vi "Shox-Total Pulse Width.vi"(1 "Shox":T1={"Rate (pps)"=0.0, "Polarity"=enum."POS", "dB Attenuation"=0.0, "Mode"=enum."Free Run", "Duration (ms)"=0.0, "Burst rate (Hz)"=0.0, "Pulse width (us)"=0.0, "Offset (ms)"=0.0, "Persist"=FALSE, "Sync"=FALSE}) -> (0 "Total pulse width (ms)":dbl)   [LabVIEW 2020]
uses:
  Cochlear Function Test Suite/LV Source/Measurement Sequence VIs/TypeDefs/Pulse Params XCtl/Data.ctl
  Pulse Polarity.ctl
  Cochlear Function Test Suite/LV Source/Measurement Sequence VIs/TypeDefs/Pulse Params XCtl/Shox Mode Enum.ctl
  Cochlear Function Test Suite/LV Source/Measurement Sequence VIs/TypeDefs/Pulse Params XCtl/MS-Pulse Params.xctl
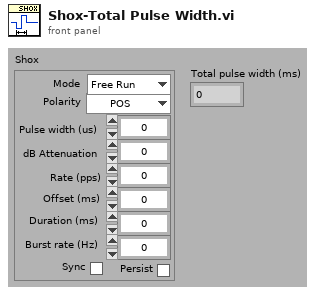
[diagram p1: front panel]
types:
  T1 = typedef "MS-Pulse Params.xctl/Data.ctl" = cluster{"Rate (pps)":dbl, "Polarity":T2, "dB Attenuation":dbl, "Mode":T3, "Duration (ms)":dbl, "Burst rate (Hz)":dbl, "Pulse width (us)":dbl, "Offset (ms)":dbl, "Persist":bool, "Sync":bool}
  T2 = typedef "Pulse Polarity.ctl" = enum16{"POS", "NEG", "POS-NEG", "NEG-POS"}
  T3 = typedef "Shox Mode Enum.ctl" = enum16{"OFF", "Free Run", "Bursted"}
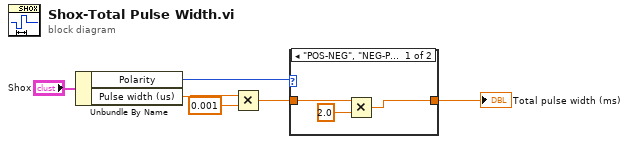
[diagram p0: block diagram]
diagram:
  n1 = Unbundle By Name("Shox") -> ("Polarity"=w4:T2, "Pulse width (us)"=w3:dbl)
  n2 = Multiply(x=w3, y=0.001) -> (x*y=w2:dbl)
  n3 = case shown="\"POS-NEG\", \"NEG-POS\", Default" w4 {
    tunnel: w2 -> [w9 w10]
    tunnel: [w7 w10] -> w1
    frame "POS-NEG", "NEG-POS", Default {
      n4 = Multiply(x=w9, y=2.0) -> (x*y=w7:dbl)
    }
    frame "POS", "NEG" {
    }
  }
  "Total pulse width (ms)" <- w1
